vi "__GetStatsLadder.vi"(8 "error in (no error)":errorcluster, 11 "ClashRoyale in":refnum<class "StashRoyale.lvclass">) -> (0 "error out":errorcluster, 3 "ClashRoyale out":refnum<class "StashRoyale.lvclass">)   [LabVIEW 2020, in "StashRoyale.lvclass"]
uses:
  StashRoyale.lvclass
  StashRoyale.lvclass/StashRoyale.ctl
panel:
  out "Extracted Section":string[](array[string])
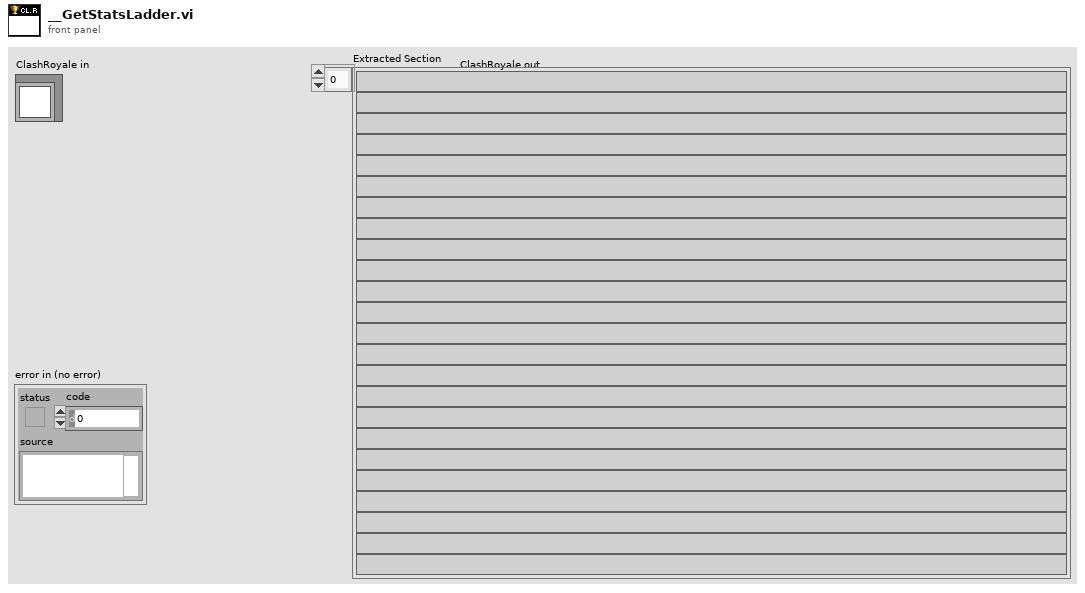
[diagram p1: front panel]
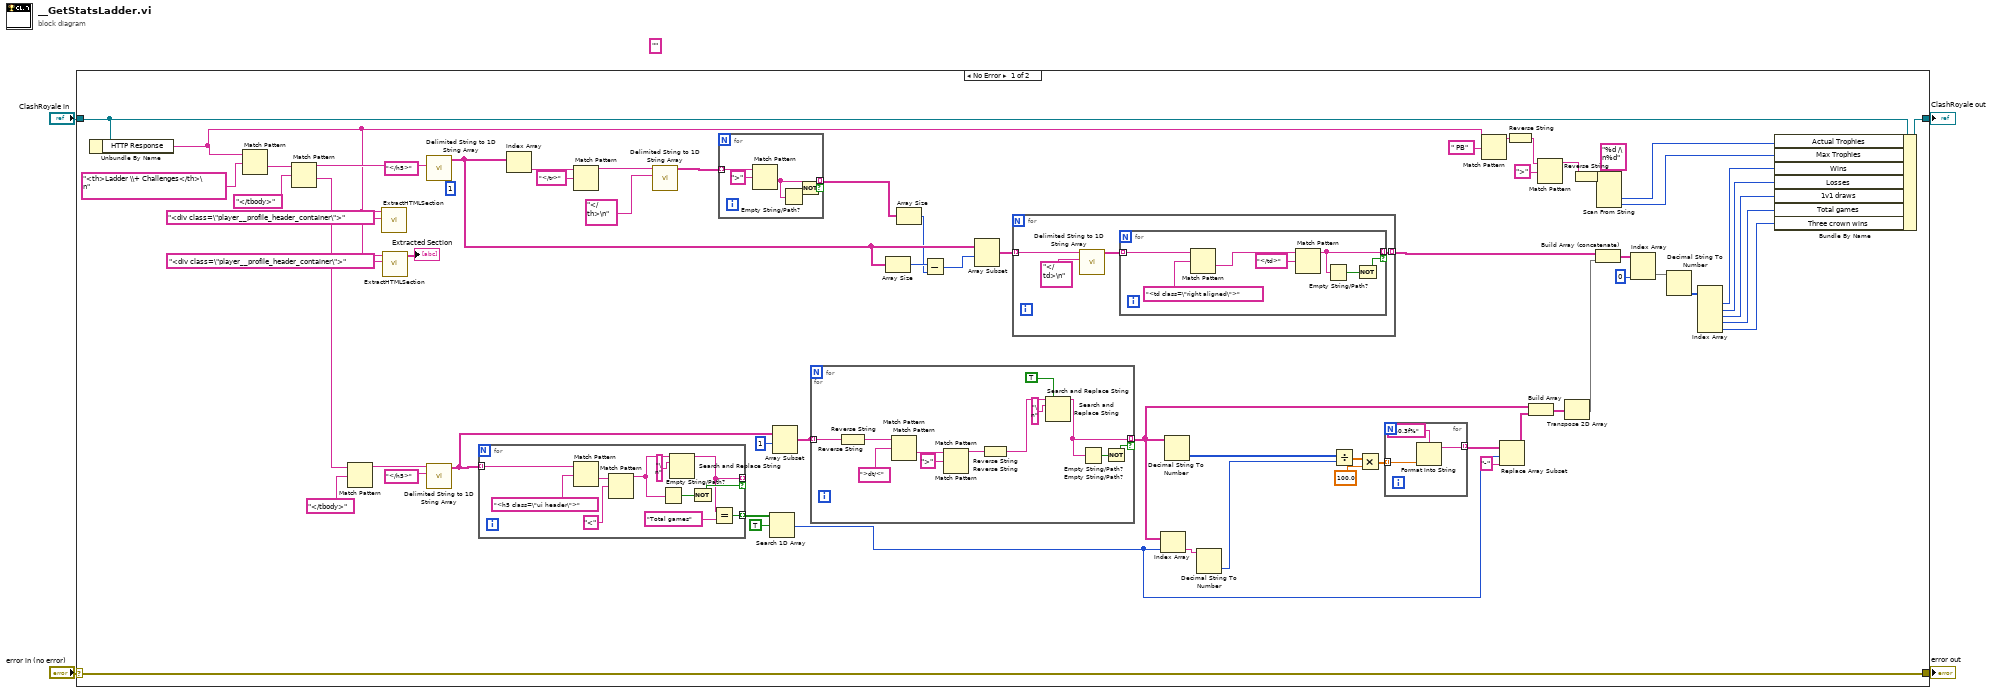
[diagram p0: block diagram]
diagram:
  (unwired) ""
  n1 = case shown="No Error" "error in (no error)" {
    selector: "error in (no error)" -> [w68 w124]
    tunnel: [w68 w124] -> w3
    tunnel: [w27 w123] -> w1
    tunnel: "ClashRoyale in" -> [w28 w123]
    frame No Error {
      (unwired) 1 ("index")
      n2 = Unbundle By Name(w28) -> ("HTTP Response"=w7:string)
      n3 = Match Pattern(string=w7, regular expression="<th>Ladder \\+ Challenges</th>\n") -> (after substring=w63:string)  [unwired: 1 in, 3 out]
      n4 = Match Pattern(string=w63, regular expression="</tbody>") -> (before substring=w60:string, after substring=w51:string)  [unwired: 1 in, 2 out]
      n5 = Match Pattern(string=w51, regular expression="</tbody>") -> (before substring=w54:string)  [unwired: 1 in, 3 out]
      n6 = call "ExtractHTMLSection.vi"("Section"="<div class=\"player__profile_header_container\">" ("Section to find"), "HTMLString"=w7) -> ()  [unwired: 9 in, 1 out]
      n7 = call "ExtractHTMLSection.vi"("Section"="<div class=\"player__profile_header_container\">", "HTMLString"=w7) -> ("Extracted Section"=→"Extracted Section":string[])  [unwired: 9 in]
      n8 = call <vilib>:"Delimited String to 1D String Array.vi"("delimiter"="</h5>", "delimited string"=w60) -> ("string array"=w58:string[])  [unwired: 9 in]
      n9 = call <vilib>:"Delimited String to 1D String Array.vi"("delimiter"="</h5>", "delimited string"=w54) -> ("string array"=w50:string[])  [unwired: 9 in]
      n10 = for {
        tunnel: w50 -> [w105] mode=indexing
        tunnel: [w98] -> _ mode=indexing if=w103
        tunnel: [w96] -> w37 mode=indexing
        n11 = Match Pattern(string=w105, regular expression="<h5 class=\"ui header\">") -> (after substring=w102:string)  [unwired: 1 in, 3 out]
        n12 = Match Pattern(string=w102, regular expression="<") -> (before substring=w100:string)  [unwired: 1 in, 3 out]
        n13 = Empty String/Path?(string/path=w100) -> (empty?=w104:bool)
        n14 = Search and Replace String(input string=w100, search string="\n") -> (result string=w98:string)  [unwired: 6 in, 3 out]
        n15 = Not(x=w104) -> (.not. x?=w103:bool)
        n16 = Equal?(x=w98, y="Total games") -> (x = y?=w96:bool)
      }
      n17 = Index Array(array=w58) -> (element=w59:string)  [unwired: 1 in]
      n18 = Match Pattern(string=w59, regular expression="</tr>") -> (before substring=w65:string)  [unwired: 1 in, 3 out]
      n19 = call <vilib>:"Delimited String to 1D String Array.vi"("delimiter"="</th>\n", "delimited string"=w65) -> ("string array"=w64:string[])  [unwired: 9 in]
      n20 = for {
        tunnel: w64 -> [w122] mode=indexing
        tunnel: [w120] -> w55 mode=indexing if=w118
        n21 = Match Pattern(string=w122, regular expression=">") -> (after substring=w120:string)  [unwired: 1 in, 3 out]
        n22 = Empty String/Path?(string/path=w120) -> (empty?=w119:bool)
        n23 = Not(x=w119) -> (.not. x?=w118:bool)
      }
      n24 = Search 1D Array(1D array=w37, element=TRUE) -> (index of element=w32:i32)  [unwired: 1 in]
      n25 = Array Subset(array=w50, index=1) -> (w30:string[])  [unwired: 1 in]
      n26 = for {
        tunnel: w30 -> [w72] mode=indexing
        tunnel: [w80] -> _ mode=indexing if=w71
        n27 = Reverse String(1:w72) -> (0:w70:string)
        n28 = Match Pattern(string=w70, regular expression=">dt/<") -> (after substring=w77:string)  [unwired: 1 in, 3 out]
        n29 = Match Pattern(string=w77, regular expression=">") -> (before substring=w74:string)  [unwired: 1 in, 3 out]
        n30 = Reverse String(1:w74) -> (0:w69:string)
        n31 = Search and Replace String(replace all?=TRUE ("replace all? (F)"), input string=w69, search string="\n") -> (result string=w80:string)  [unwired: 5 in, 3 out]
        n32 = Empty String/Path?(string/path=w80) -> (empty?=w76:bool)
        n33 = Not(x=w76) -> (.not. x?=w71:bool)
      }
      n34 = for {
        tunnel: w30 -> [w87] mode=indexing
        tunnel: [w95] -> w35 mode=indexing if=w86
        n35 = Reverse String(1:w87) -> (0:w85:string)
        n36 = Match Pattern(string=w85, regular expression=">dt/<") -> (after substring=w92:string)  [unwired: 1 in, 3 out]
        n37 = Match Pattern(string=w92, regular expression=">") -> (before substring=w89:string)  [unwired: 1 in, 3 out]
        n38 = Reverse String(1:w89) -> (0:w84:string)
        n39 = Search and Replace String(replace all?=TRUE ("replace all? (F)"), input string=w84, search string="\n") -> (result string=w95:string)  [unwired: 5 in, 3 out]
        n40 = Empty String/Path?(string/path=w95) -> (empty?=w91:bool)
        n41 = Not(x=w91) -> (.not. x?=w86:bool)
      }
      n42 = Array Size(array=w58) -> (size(s)=w57:i32)
      n43 = Array Size(array=w55) -> (size(s)=w48:i32)
      n44 = Subtract(x=w57, y=w48) -> (x-y=w56:i32)
      n45 = Array Subset(array=w58, index=w56) -> (w29:string[])  [unwired: 1 in]
      n46 = for {
        tunnel: w29 -> [w109] mode=indexing
        tunnel: [w107] -> w46 mode=indexing
        n47 = call <vilib>:"Delimited String to 1D String Array.vi"("delimiter"="</td>\n", "delimited string"=w109) -> ("string array"=w108:string[])  [unwired: 9 in]
        n48 = for {
          tunnel: w108 -> [w114] mode=indexing
          tunnel: [w112] -> w107 mode=indexing if=w111
          n49 = Match Pattern(string=w114, regular expression="<td class=\"right aligned\">") -> (after substring=w115:string)  [unwired: 1 in, 3 out]
          n50 = Match Pattern(string=w115, regular expression="</td>") -> (before substring=w112:string)  [unwired: 1 in, 3 out]
          n51 = Empty String/Path?(string/path=w112) -> (empty?=w113:bool)
          n52 = Not(x=w113) -> (.not. x?=w111:bool)
        }
      }
      n53 = Index Array(array=w35, index=w32) -> (element=w45:string)
      n54 = Decimal String To Number(string=w35) -> (number=w44:i32[])  [unwired: 2 in, 1 out]
      n55 = Decimal String To Number(string=w45) -> (number=w34:i32)  [unwired: 2 in, 1 out]
      n56 = Divide(x=w44, y=w34) -> (x/y=w43:dbl[])
      n57 = Multiply(x=w43, y=100.0) -> (x*y=w41:dbl[])
      n58 = for {
        tunnel: w41 -> [w83] mode=indexing
        tunnel: [w81] -> w40 mode=indexing
        n59 = Format Into String(format string="%0.3f%", w83) -> (resulting string=w81:string)  [unwired: 2 in, 1 out]
      }
      n60 = Match Pattern(string=w7, regular expression=" PB") -> (before substring=w16:string)  [unwired: 1 in, 3 out]
      n61 = Replace Array Subset(array=w40, new element="-" ("new element/subarray"), index=w32) -> (w33:string[])
      n62 = Reverse String(1:w16) -> (0:w13:string)
      n63 = Build Array(w35, w33) -> (w39:string[][])
      n64 = Match Pattern(string=w13, regular expression=">") -> (before substring=w12:string)  [unwired: 1 in, 3 out]
      n65 = Transpose 2D Array(2D array=w39) -> (transposed array=w38:string[][])
      n66 = Reverse String(1:w12) -> (0:w11:string)
      n67 = Build Array (concatenate)(w46, w38) -> (w26:string[][])
      n68 = Scan From String(format string="%d /\n%d", input string=w11) -> (output 1=w10:i32, output 2=w9:i32)  [unwired: 4 in, 3 out]
      n69 = Index Array(array=w26, index (col)=0 ("disabled index (col)")) -> (element=w24:string[])  [unwired: 1 in]
      n70 = Decimal String To Number(string=w24) -> (number=w23:i32[])  [unwired: 2 in, 1 out]
      n71 = Index Array(array=w23) -> (element #1=w22:i32, element #2=w21:i32, element #3=w20:i32, element #4=w19:i32, element #5=w18:i32)  [unwired: 5 in]
      n72 = Bundle By Name(cluster=w28, "Actual Trophies"=w10, "Max Trophies"=w9, "Wins"=w22, "Losses"=w21, "1v1 draws"=w20, "Total games"=w19, "Three crown wins"=w18) -> (w27:refnum<class "StashRoyale.lvclass">)
    }
    frame Error {
    }
  }
  "error out" <- w3
  "ClashRoyale out" <- w1
